vi "Add To Profile.vi"(8 "error in (no error)":errorcluster, 10 "Pofil":string, 11 "Output Actor Hardware in":refnum<class "Output Actor Hardware.lvclass">) -> (0 "error out":errorcluster, 3 "Output Actor Hardware out":refnum<class "Output Actor Hardware.lvclass">)   [LabVIEW 2015, in "Output Actor Hardware.lvclass"]
uses:
  Output Actor Hardware.lvclass
  Output Actor Hardware.lvclass/Output Actor Hardware.ctl
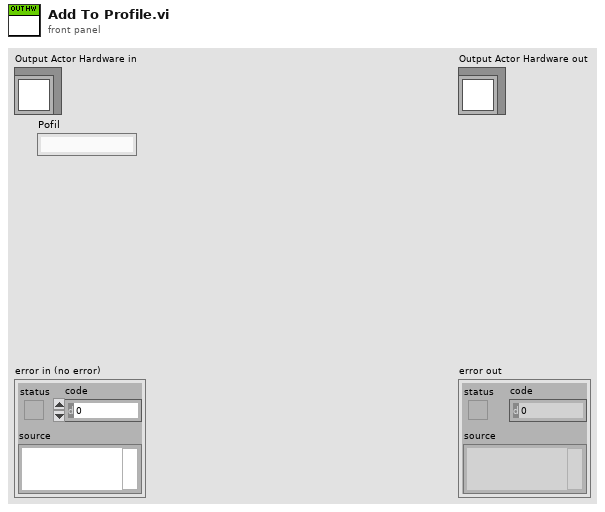
[diagram p1: front panel]
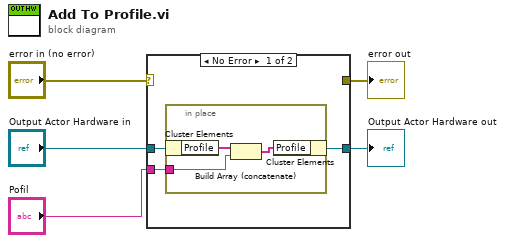
[diagram p0: block diagram]
diagram:
  n1 = case shown="No Error" "error in (no error)" {
    selector: "error in (no error)" -> [_ w13]
    tunnel: [_ w13] -> w4
    tunnel: [w7 w12] -> w2
    tunnel: "Output Actor Hardware in" -> [w8 w12]
    tunnel: "Pofil" -> [w6 _]
    frame No Error {
      n2 = in-place {
        in-place-border: w6 -> [w9]
        n3 = in-place-cluster #1(w8) -> ("Profile"=w11:string[])
        n4 = Build Array (concatenate)(w11, w9) -> (w10:string[])
        n5 = in-place-cluster #1("Profile"=w10) -> (w7:refnum<class "Output Actor Hardware.lvclass">)
      }
    }
    frame Error {
    }
  }
  "error out" <- w4
  "Output Actor Hardware out" <- w2
